vi "configure operation.vi"(7 "tag bus configurable plugin module configuration":refnum<class "UI Reference configuration.lvclass">=refnum, 8 "error in":errorcluster, 10 "line item in":T2, 11 "engine configuration":refnum<class "engine configuration.lvclass">) -> (0 "error out":errorcluster, 1 "success":bool, 2 "line item out":T2, 5 "changed":bool)   [LabVIEW 2014, in "UI Reference editor node.lvclass"]
uses:
  UI Reference editor node.lvclass
  <vilib>/NI/Tag Bus/tag/tag descriptor.lvclass
  <vilib>/NI/Module Execution Interface/Engine Configuration/engine configuration.lvclass
  module/configuration/UI Reference configuration.lvclass
  <vilib>/NI/Tag Bus Module Framework/channel/TBM channel.lvclass
  table line.ctl
  permissions.ctl
panel:
  out "errors":string
  in  "Access Type":T1
  in  "Tag":i32(listbox)
  in  "Data Type":i32(listbox)
  in  "Terminal Label":string
  in  "cancel":bool
  in  "ok":bool
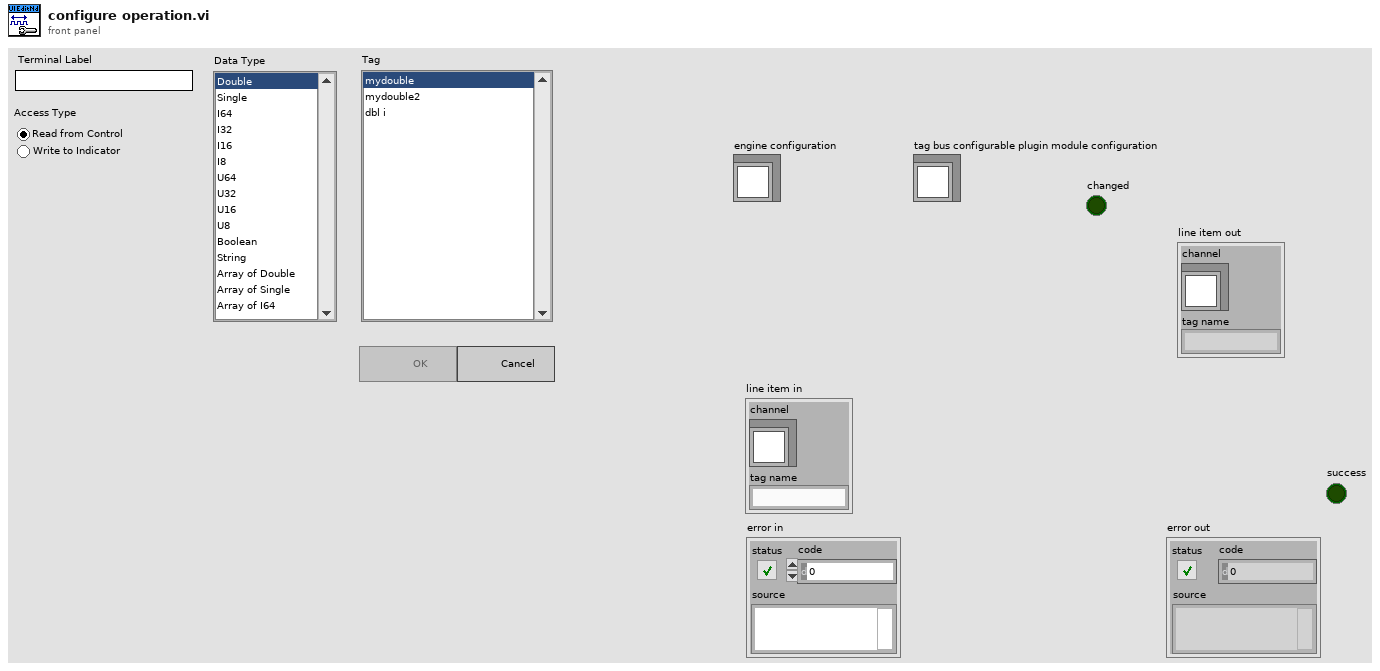
[diagram p1: front panel]
types:
  T1 = typedef "UI Reference editor node.lvclass/permissions.ctl" = enum32{"Read from Control", "Write to Indicator"}
  T2 = typedef "UI Reference editor node.lvclass/table line.ctl" = cluster{"channel":refnum<class "TBM channel.lvclass">, "tag name":string}
  T3 = enum32{"Invalid", "Standard", "Closed", "Hidden", "Minimized", "Maximized"}
  T4 = enum32{"Invalid", "Default", "Floating", "Floating/Auto-Hide", "Modal"}
  T5 = enum8{"Enabled", "Disabled", "Disabled and Grayed Out"}
  T6 = enum32{"invalid app kind", "Development System", "Run Time System", "Student Edition", "Embedded LabVIEW", "Evaluation", "Custom"}
  T7 = typedef "TBM channel.lvclass/channel classification.ctl" = enum16{"input data", "output data", "processing parameter", "processing result"}
  T8 = typedef "tag bus.lvlib/tag descriptor.lvclass/Data Type.ctl" = enum16{"Double", "Single", "I64", "I32", "I16", "I8", "U64", "U32", "U16", "U8", "Boolean", "String", "Array of Double", "Array of Single", "Array of I64", "Array of I32", "Array of I16", "Array of I8", "Array of U64", "Array of U32", "Array of U16", "Array of U8", "Array of Boolean", "Array of String"}
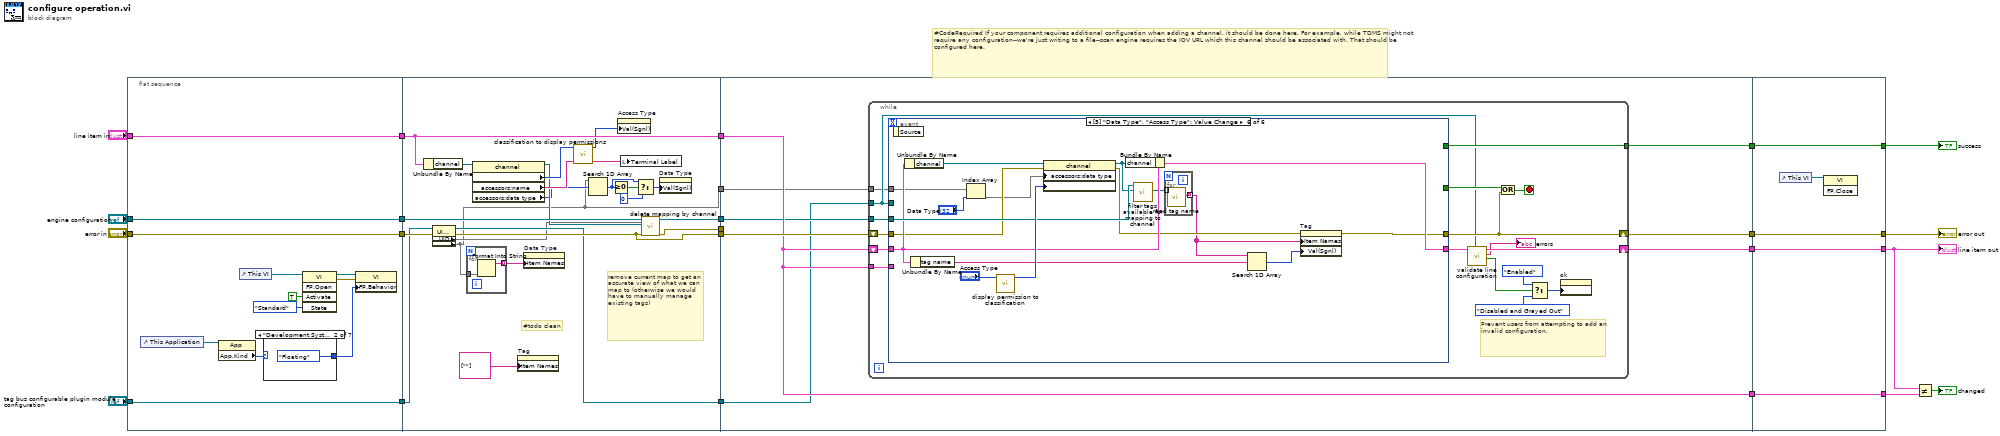
[diagram p0: block diagram]
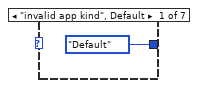
[diagram p2: hidden frame]
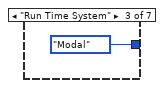
[diagram p3: hidden frame]
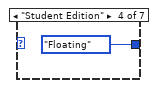
[diagram p4: hidden frame]
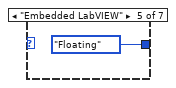
[diagram p5: hidden frame]
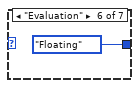
[diagram p6: hidden frame]
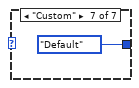
[diagram p7: hidden frame]
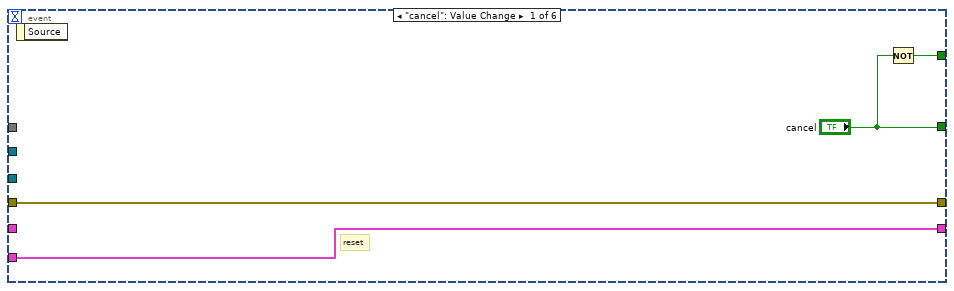
[diagram p8: hidden frame]
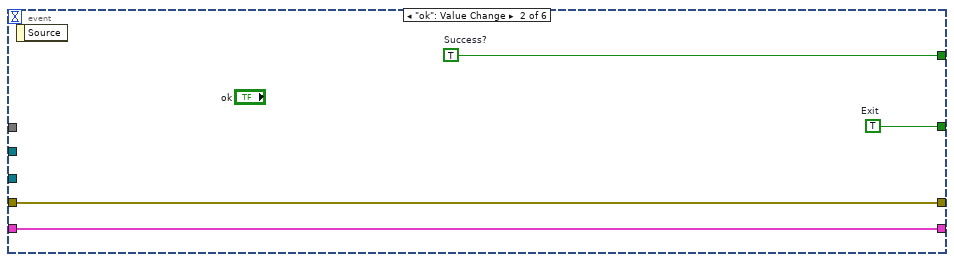
[diagram p9: hidden frame]
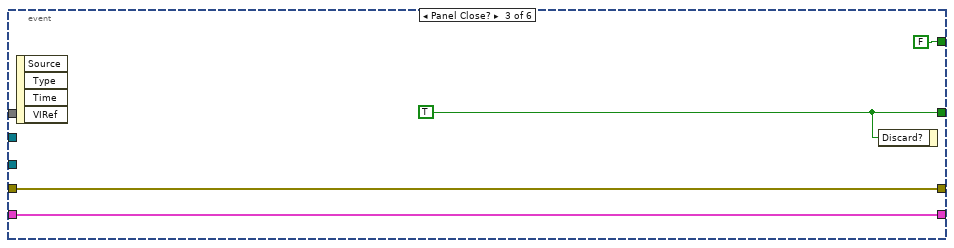
[diagram p10: hidden frame]
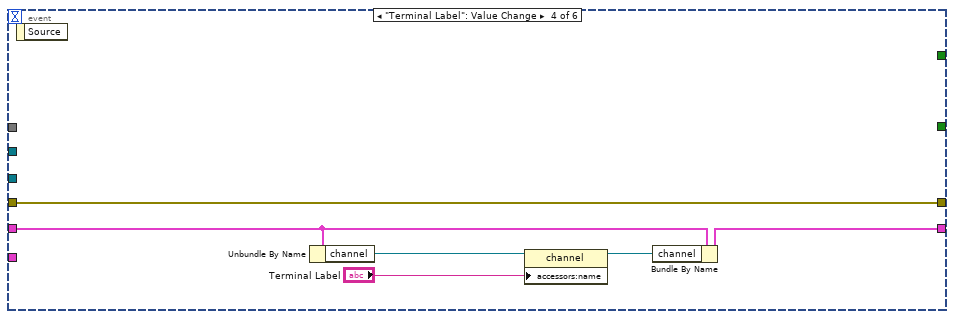
[diagram p11: hidden frame]
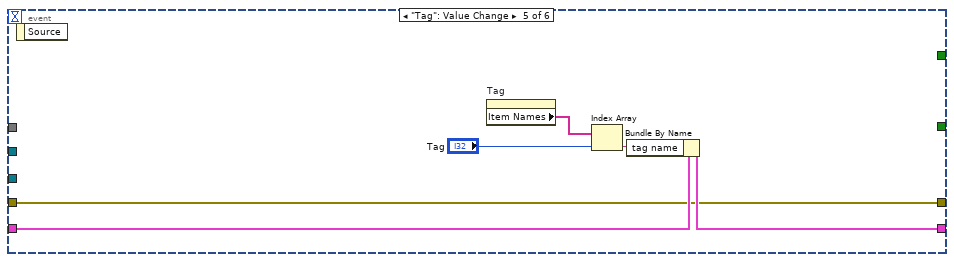
[diagram p12: hidden frame]
diagram:
  # "#CodeRequired If your component requires additional configuration when adding a channel, it should be done here. For example, while TDMS might not require any configuration--we're just writing to a file--scan engine requires the IOV URL which this channel should be associated with. That should be configured here."
  n1 = flat-sequence {
    tunnel: "line item in" -> [w34]
    tunnel: "error in" -> [w35]
    tunnel: [w35] -> w12
    tunnel: [w34] -> w11
    tunnel: [w25] -> w8
    tunnel: "engine configuration" -> [w25]
    tunnel: [w24] -> w5
    tunnel: "tag bus configurable plugin module configuration" -> [w24]
    tunnel: w12 -> [w56]
    tunnel: w11 -> [w61]
    tunnel: [w61] -> w10
    tunnel: [w59] -> w9
    tunnel: w8 -> [w60]
    tunnel: [w53] -> w6
    tunnel: w5 -> [w54]
    tunnel: [w55] -> w3
    tunnel: [w57] -> w2
    tunnel: [w43] -> w1
    tunnel: [w73] -> w16
    tunnel: [w72] -> w15
    tunnel: [w71] -> w14
    tunnel: [w70] -> w13
    tunnel: w10 -> [w70]
    tunnel: w9 -> [w69]
    tunnel: w6 -> [w68]
    tunnel: w3 -> [w74]
    tunnel: w2 -> [_]
    tunnel: w1 -> [w67]
    tunnel: [w136] -> w17
    tunnel: [w137] -> w20
    tunnel: [w138] -> w21
    tunnel: [w139] -> w22
    tunnel: w16 -> [w139]
    tunnel: w15 -> [w138]
    tunnel: w14 -> [w137]
    tunnel: w13 -> [w136]
    frame #0 {
      n2 = control-ref of="This Application"() -> (w28:refnum<vi>)
      n3 = property class="App"(reference=w28) -> ("App.Kind"=w27:T6)  [unwired: 1 in, 2 out]
      n4 = control-ref of="This VI"() -> (w29:refnum<vi>)
      n5 = case shown="\"Development System\"" w27 {
        tunnel: [T4."Default" ("Front Panel Window:Behavior") T4."Floating" ("Front Panel Window:Behavior") T4."Modal" ("Front Panel Window:Behavior") T4."Floating" ("Front Panel Window:Behavior") T4."Floating" ("Front Panel Window:Behavior") T4."Floating" ("Front Panel Window:Behavior") T4."Default" ("Front Panel Window:Behavior")] -> w26
        frame "invalid app kind", Default {
        }
        frame "Development System" {
        }
        frame "Run Time System" {
        }
        frame "Student Edition" {
        }
        frame "Embedded LabVIEW" {
        }
        frame "Evaluation" {
        }
        frame "Custom" {
        }
      }
      n6 = invoke class="VI" method="FP.Open"(reference=w29, "Activate"=TRUE ("Activate?"), "State"=T3."Standard") -> (reference out=w32:refnum<vi>, error out=w33:errorcluster)  [unwired: 2 in, 3 out]
      n7 = property class="VI"(reference=w32, error in=w33, "FP.Behavior"=w26) -> ()  [unwired: 2 out]
    }
    frame #1 {
      # "#todo clean"
      # "remove current map to get an accurate view of what we can map to (otherwise we would have to manually manage existing tags)"
      n8 = Unbundle By Name(w61) -> ("channel"=w62:refnum<class "TBM channel.lvclass">)
      n9 = property class="UI Reference configuration.lvcl"(reference=w54, error in=w56) -> (reference out=w53:refnum<class "UI Reference configuration.lvclass">, error out=w55:errorcluster, "Properties:UID"=w52, "Properties:supported types"=w43)
      n10 = for {
        tunnel: w43 -> [w66]
        tunnel: [w65] -> w51 mode=indexing
        n11 = Format Into String(w66) -> (resulting string=w65:string)  [unwired: 3 in, 1 out]
      }
      n12 = property class="channel"(reference=w62) -> (reference out=w58:refnum<class "TBM channel.lvclass">, "data access:channel classification"=w64:T7, "accessors:name"=w63:string, "accessors:data type"=w44:T8)  [unwired: 1 in, 1 out]
      n13 = property on="Tag" class="LstBox (strict)"("Item Names"=string[] [""]) -> ()  [unwired: 2 in, 2 out]
      n14 = property on="Data Type" class="LstBox (strict)"("Item Names"=w51) -> ()  [unwired: 2 in, 2 out]
      n15 = call "classification to display permissions.vi"("channel classification"=w64) -> ("permissions"=w45:T1)  [unwired: 10 in]
      n16 = Search 1D Array(1D array=w43, element=w44) -> (index of element=w49:i32)  [unwired: 1 in]
      n17 = Greater Or Equal To 0?(x=w49) -> (x >= 0?=w50:bool)
      n18 = property on="Access Type" class="RadioBtnsControl (strict)"("Val(Sgnl)"=w45) -> ()  [unwired: 2 in, 2 out]
      n19 = local write "Terminal Label"(w63) -> ()
      n20 = Select(t=w49, s=w50, f=0) -> (s? t:f=w47:i32)
      n21 = call <vilib>:"delete mapping by channel.vi"("owner ID"=w52, "error in"=w55, "channel"=w58, "engine configuration in"=w60) -> ("error out"=w57:errorcluster, "engine configuration out"=w59:refnum<class "engine configuration.lvclass">)  [unwired: 6 in]
      n22 = property on="Data Type" class="LstBox (strict)"("Val(Sgnl)"=w47) -> ()  [unwired: 2 in, 2 out]
    }
    frame #2 {
      n23 = while {
        shift-right: [w82] -> w72
        shift-left: w74 -> [w90]
        tunnel: [w89] -> w73
        shift-right: [w83] -> w71
        shift-left: w70 -> [w86]
        tunnel: w70 -> [w85]
        tunnel: w69 -> [w91]
        tunnel: w68 -> [w77]
        tunnel: w67 -> [w76]
        stop <- w87 stop-if-true
        # "Prevent users from attempting to add an invalid configuration."
        n24 = event shown="[5] \"Data Type\", \"Access Type\": Value Change" {
          selector: _ -> [_ _ _ _ _ _]
          dyn-events: _ -> [_ _ _ _ _ _]
          timeout: _ -> [_ _ _ _ _ _]
          tunnel: w91 -> [_ _ _ _ _ w130]
          tunnel: w90 -> [w95 w99 w103 w109 w112 w123]
          tunnel: [w95 w99 w103 w109 w112 w118] -> w82
          tunnel: [w94 w96 FALSE _ _ _] -> w89
          tunnel: ["cancel" w97 w101 _ _ _] -> w88
          tunnel: w86 -> [_ w98 w100 w107 w115 w128]
          tunnel: [w92 w98 w100 w108 w114 w127] -> w84
          tunnel: w85 -> [w92 _ _ _ _ _]
          tunnel: w77 -> [_ _ _ _ _ _]
          tunnel: w76 -> [_ _ _ _ _ w122]
          event "cancel": Value Change {
            # "reset"
            n25 = event-data() -> ()  [unwired: 1 in, 1 out]
            n26 = Not(x="cancel") -> (.not. x?=w94:bool)
          }
          event "ok": Value Change {
            w96 = TRUE  # Success?
            w97 = TRUE  # Exit
            n27 = event-data() -> ()  [unwired: 1 in, 1 out]
          }
          event Panel Close? {
            w101 = TRUE ("cancel")
            n28 = event-data() -> ()  [unwired: 1 in, 4 out]
            n29 = event-data("Discard?"=w101) -> ()  [unwired: 1 in, 1 out]
          }
          event "Terminal Label": Value Change {
            n30 = event-data() -> ()  [unwired: 1 in, 1 out]
            n31 = Unbundle By Name(w107) -> ("channel"=w106:refnum<class "TBM channel.lvclass">)
            n32 = property class="channel"(reference=w106, "accessors:name"="Terminal Label") -> (reference out=w105:refnum<class "TBM channel.lvclass">)  [unwired: 1 in, 1 out]
            n33 = Bundle By Name(cluster=w107, "channel"=w105) -> (w108:T2)
          }
          event "Tag": Value Change {
            n34 = event-data() -> ()  [unwired: 1 in, 1 out]
            n35 = property on="Tag" class="LstBox (strict)"() -> ("Item Names"=w110:string[])  [unwired: 2 in, 2 out]
            n36 = Index Array(array=w110, index="Tag") -> (element=w113:string)
            n37 = Bundle By Name(cluster=w115, "tag name"=w113) -> (w114:T2)
          }
          event "Data Type": Value Change {
            n38 = event-data() -> ()  [unwired: 1 in, 1 out]
            n39 = Unbundle By Name(w128) -> ("channel"=w132:refnum<class "TBM channel.lvclass">)
            n40 = Unbundle By Name(w128) -> ("tag name"=w125:string)
            n41 = Index Array(array=w122, index="Data Type") -> (element=w120)
            n42 = call "display permission to classification.vi"("display permissions"="Access Type") -> ("channel classification"=w131:T7)  [unwired: 10 in]
            n43 = property class="channel"(reference=w132, error in=w123, "accessors:data type"=w120, "data access:channel classification"=w131) -> (reference out=w129:refnum<class "TBM channel.lvclass">, error out=w119:errorcluster)
            n44 = Bundle By Name(cluster=w128, "channel"=w129) -> (w127:T2)
            n45 = call-dynamic "filter tags available for mapping to channel.vi"("channel to map to"=w129, "engine configuration in"=w130) -> ("filtered tags"=w126:refnum<class "tag descriptor.lvclass">[])  [unwired: 8 in, 1 out]
            n46 = for {
              tunnel: w126 -> [w134] mode=indexing
              tunnel: [w133] -> w117 mode=indexing
              n47 = call <vilib>:"read tag name.vi"("system tag in"=w134) -> ("name"=w133:string)  [unwired: 8 in, 2 out]
            }
            n48 = Search 1D Array(1D array=w117, element=w125) -> (index of element=w116:i32)  [unwired: 1 in]
            n49 = property on="Tag" class="LstBox (strict)"(error in=w119, "Item Names"=w117, "Val(Sgnl)"=w116) -> (error out=w118:errorcluster)  [unwired: 1 in, 1 out]
          }
        }
        n50 = call "validate line configuration.vi"("module"=w77, "line in"=w84) -> ("valid?"=w81:bool, "errors"=→"errors":string, "line out"=w83:T2)  [unwired: 7 in]
        n51 = Compound Arithmetic op=OR(w88, w82) -> (w87:bool)
        n52 = Select(t=T5."Enabled" ("Disabled"), s=w81, f=T5."Disabled and Grayed Out") -> (s? t:f=w78:T5)
        n53 = property on="ok" class="Bool"("DisabledEnum"=w78) -> ()  [unwired: 2 in, 2 out]
      }
    }
    frame #3 {
      n54 = control-ref of="This VI"() -> (w135:refnum<vi>)
      n55 = invoke class="VI" method="FP.Close"(reference=w135) -> ()  [unwired: 2 in, 3 out]
    }
  }
  n56 = Not Equal?(x=w20, y=w17) -> (x != y?=→"changed":bool)
  "error out" <- w21
  "success" <- w22
  "line item out" <- w20
